vi "Exercise 2- Acquire.vi"() -> ()   [LabVIEW 2012]
panel:
  out "Filtered Signal":dynamicdata(graph)
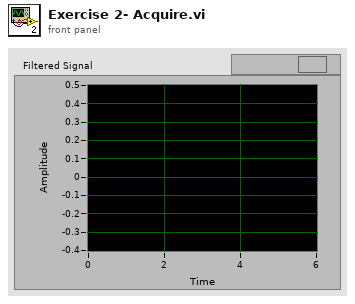
[diagram p1: front panel]
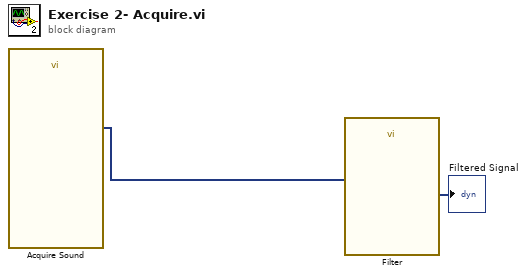
[diagram p0: block diagram]
diagram:
  n1 = call "Acquire Sound"() -> ("Data"=w2:dynamicdata)  [unwired: 18 in, 1 out]
  n2 = call "Filter"("Signal"=w2) -> ("Filtered Signal"=→"Filtered Signal":dynamicdata)  [unwired: 9 in, 1 out]
